vi "Save Data From Acquisition Temp File.vi"(8 "error in":errorcluster, 9 "Type":string="Arrival Time Counter", 10 "Arrival Time Temp File":refnum<file>, 11 "refnum in":refnum<file>) -> (0 "error out":errorcluster, 3 "refnum":refnum<file>)   [LabVIEW 2009]
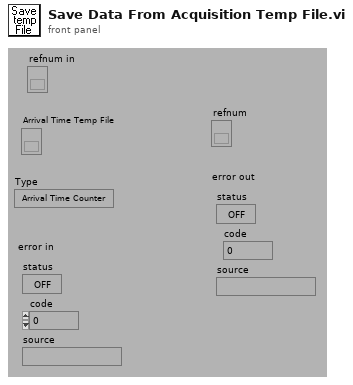
[diagram p1: front panel]
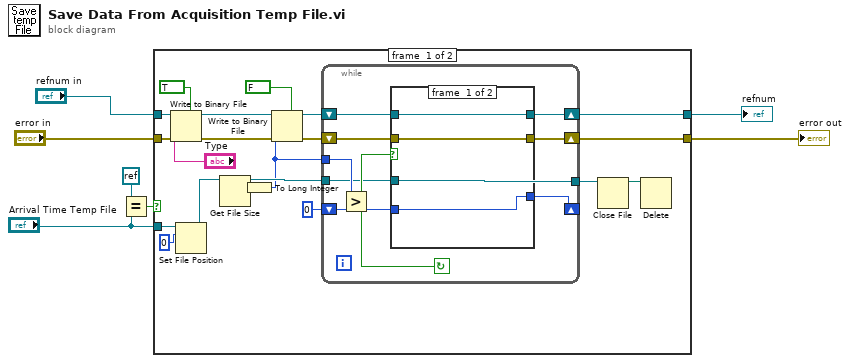
[diagram p0: block diagram]
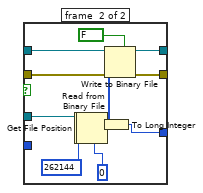
[diagram p2: hidden frame]
diagram:
  n1 = Equal?(x=refnum<k0> refnum, y="Arrival Time Temp File") -> (x = y?=w1:bool)
  n2 = case shown="False" w1 {
    tunnel: "refnum in" -> [w24 w54]
    tunnel: [w27 w54] -> w5
    tunnel: [w26 w53] -> w6
    tunnel: "error in" -> [w25 w53]
    tunnel: "Arrival Time Temp File" -> [w12 _]
    frame #0 {
      n3 = Write to Binary File(file (use dialog)=w24, data="Type", error in=w25, 5:TRUE ("header (F)")) -> (refnum out=w23:refnum<file>, error out=w22:errorcluster)  [unwired: 2 in, 1 out]
      n4 = Set File Position(offset (in bytes) (0)=0 ("pos offset (0)"), refnum=w12) -> (refnum out=w11:refnum<file>)  [unwired: 2 in, 1 out]
      n5 = Get File Size(file=w11) -> (refnum out=w17:refnum<file>, size (in bytes)=w8:i64)  [unwired: 1 in, 1 out]
      n6 = To Long Integer(number=w8) -> (32bit integer=w14:i32)
      n7 = Write to Binary File(file (use dialog)=w23, data=w14, error in=w22, 5:FALSE ("prepend array or string size? (T)")) -> (refnum out=w15:refnum<file>, error out=w16:errorcluster)  [unwired: 2 in, 1 out]
      n8 = while {
        tunnel: [w34] -> w21
        tunnel: w17 -> [w34]
        tunnel: w14 -> [w36]
        shift-left: 0 ("offset") -> [w32]
        shift-right: [w33] -> _
        shift-left: w16 -> [w30]
        shift-right: [w29] -> w26
        shift-left: w15 -> [w31]
        shift-right: [w28] -> w27
        stop <- w35 continue-if-true
        n9 = Greater?(x=w36, y=w32) -> (0:w35:bool)
        n10 = case shown="True" w35 {
          tunnel: w34 -> [_ w52]
          tunnel: [w39 w51] -> w33
          tunnel: w32 -> [w39 _]
          tunnel: w31 -> [w38 w48]
          tunnel: w30 -> [w37 w47]
          tunnel: [w37 w46] -> w29
          tunnel: [w38 w45] -> w28
          frame #0 {
          }
          frame #1 {
            n11 = Read from Binary File(5:u8 0 ("byte stream type"), 10:262144 ("count"), 11:w52) -> (0:w42:errorcluster, 2:w49:u8[], 3:w43:refnum<file>)  [unwired: 3 in, 1 out]
            n12 = Get File Position(4:w42, 7:w43) -> (2:w41:i64)  [unwired: 2 out]
            n13 = To Long Integer(number=w41) -> (32bit integer=w51:i32)
            n14 = Write to Binary File(file (use dialog)=w48, data=w49, error in=w47, 5:FALSE ("prepend array or string size? (T)")) -> (refnum out=w45:refnum<file>, error out=w46:errorcluster)  [unwired: 2 in, 1 out]
          }
        }
      }
      n15 = Close File(refnum=w21) -> (path=w20:path)  [unwired: 1 in, 1 out]
      n16 = Delete(path (use dialog)=w20) -> ()  [unwired: 4 in, 3 out]
    }
    frame #1 {
    }
  }
  "error out" <- w6
  "refnum" <- w5
